vi "01_write_file.vi"() -> ()   [LabVIEW 2017]
panel:
  in  "text":string
  in  "file path (use dialog)":path
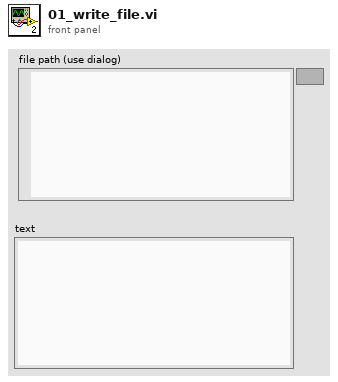
[diagram p1: front panel]
types:
  T1 = enum16{"open", "replace", "create", "open or create", "replace or create", "replace or create with confirmation"}
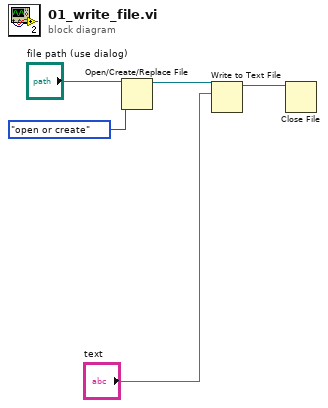
[diagram p0: block diagram]
diagram:
  n1 = Open/Create/Replace File(file path (use dialog)="file path (use dialog)", operation (0:open)=T1."open or create") -> (refnum out=w3:refnum<file>)  [unwired: 4 in, 2 out]
  n2 = Write to Text File(file (use dialog)=w3, text="text") -> (refnum out=w1:refnum<file>)  [unwired: 2 in, 2 out]
  n3 = Close File(refnum=w1) -> ()  [unwired: 1 in, 2 out]
